vi "MusicStop.vi"(8 "error in (no error)":errorcluster) -> (0 "error out":errorcluster)   [LabVIEW 2015, in "LabBASSMOD2.lvlib"]
uses:
  LabBassMOD2.lvlib
  DLL/BASSMOD.dll
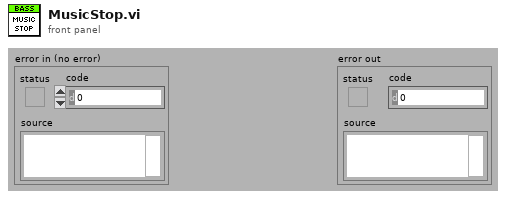
[diagram p1: front panel]
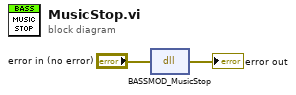
[diagram p0: block diagram]
diagram:
  n1 = dll-call lib="C:/dev/PGS/LabBASSMOD2/DLL/BASSMOD.dll" fn="BASSMOD_MusicStop"(error in="error in (no error)") -> (error out=→"error out":errorcluster)  [unwired: 3 in, 1 out]
